vi "Locked.vi"(0 "Interface in":T1, 9 "timeout (5000 ms)":i32=5000, 11 "error in":errorcluster) -> (4 "Interface out":T1, 6 "Locked":bool, 15 "error out":errorcluster)   [LabVIEW 2017, in "ThreePhasePLLInterface.lvlib"]
uses:
  ThreePhasePLLInterface.lvlib
  InterfaceRef.ctl
  <instrlib>/_niInstr/Instruction Framework/v1/Host/Instruction Target/niInstr Instruction Target v1 Host.lvclass
  <instrlib>/_niInstr/Instruction Framework/v1/Host/Instruction Framework Context/niInstr Instruction Framework Context v1 Host.lvclass
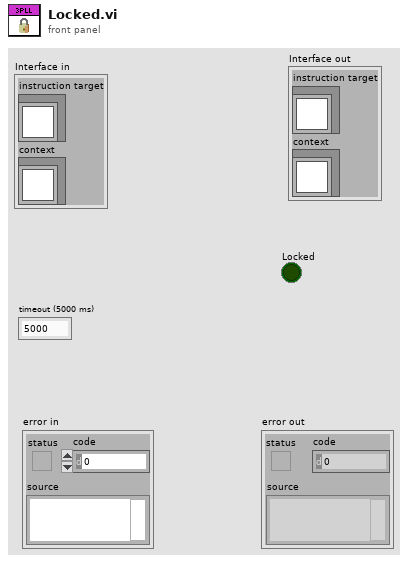
[diagram p1: front panel]
types:
  T1 = typedef "ThreePhasePLLInterface.lvlib/InterfaceRef.ctl" = cluster{"instruction target":refnum<class "niInstr Instruction Target v1 Host.lvclass">, "context":refnum<class "niInstr Instruction Framework Context v1 Host.lvclass">}
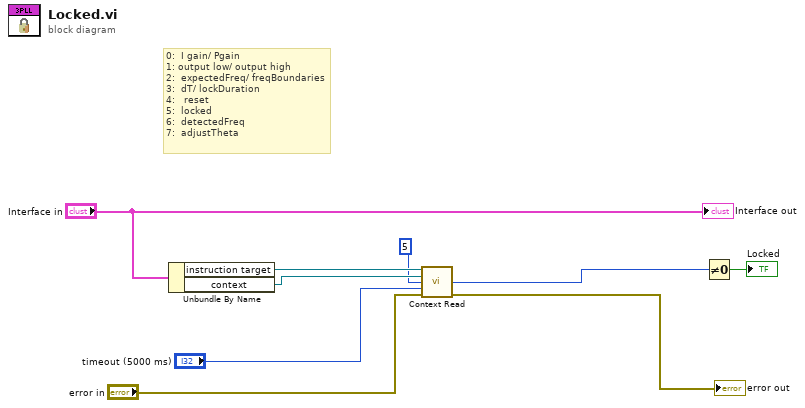
[diagram p0: block diagram]
diagram:
  # "0:  I gain/ Pgain\n1: output low/ output high\n2:  expectedFreq/ freqBoundaries\n3:  dT/ lockDuration\n4:   reset\n5:  locked\n6:  detectedFreq\n7:  adjustTheta"
  n1 = Unbundle By Name("Interface in") -> ("instruction target"=w9:refnum<class "niInstr Instruction Target v1 Host.lvclass">, "context"=w8:refnum<class "niInstr Instruction Framework Context v1 Host.lvclass">)
  n2 = call <instrlib>:"Context Read.vi"("instruction target in"=w9, "context in"=w8, "address"=u64 5, "timeout (5000 ms)"="timeout (5000 ms)", "error in"="error in") -> ("data"=w2:u64, "error out"=→"error out":errorcluster)  [unwired: 7 in, 2 out]
  n3 = Not Equal To 0?(x=w2) -> (x != 0?=→"Locked":bool)
  "Interface out" <- "Interface in"
